vi "GetElementNum.vi"(0 "input variable":i16) -> (1 "size(s)":i32, 2 "appended array":i32[](array[numeric]))   [LabVIEW 2016]
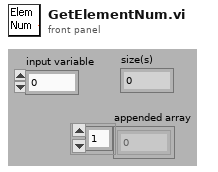
[diagram p1: front panel]
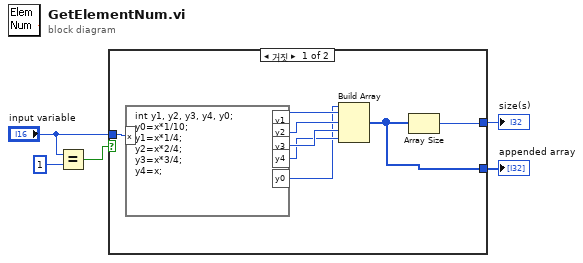
[diagram p0: block diagram]
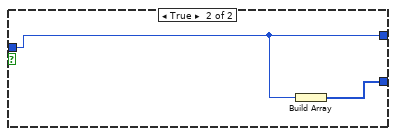
[diagram p2: hidden frame]
diagram:
  n1 = Equal?(x="input variable", y=i16 1) -> (x = y?=w2:bool)
  n2 = case shown="거짓" w2 {
    tunnel: "input variable" -> [w13 w15]
    tunnel: [w9 w15] -> w5
    tunnel: [w8 w14] -> w1
    frame False {
      n3 = formula code="int y1, y2, y3, y4, y0;\ny0=x*1/10;\ny1=x*1/4;\ny2=x*2/4;\ny3=x*3/4;\ny4=x;"("x"=w13) -> ("y1"=w12:i32, "y2"=w11:i32, "y3"=w10:i32, "y4"=w7:i32, "y0"=w6:i32)
      n4 = Build Array(w6, w12, w11, w10, w7) -> (w8:i32[])
      n5 = Array Size(array=w8) -> (size(s)=w9:i32)
    }
    frame True {
      n6 = Build Array(w15) -> (w14:i16[])
    }
  }
  "size(s)" <- w5
  "appended array" <- w1
